vi "Init.vi"(7 "Section Name":refnum<class "Section Name.lvclass">, 8 "Error In":errorcluster, 9 "Values":refnum<class "Value.lvclass">[](array[class]), 10 "Keys":refnum<class "Key Name.lvclass">[](array[class]), 11 "reference in":refnum<class "Dummy Entry.lvclass">) -> (0 "Error Out":errorcluster, 3 "reference out":refnum<class "Dummy Entry.lvclass">)   [LabVIEW 2024, in "Electronic Datasheet.lvlib" / "Dummy Entry.lvclass"]
uses:
  Dummy Entry.lvclass
  Dummy Entry.lvclass/Dummy Entry.ctl
  Object Type/Object Type Base.lvclass
  OD Entry/OD Entry.lvclass
  D:/git/EDS-File-Viewer/Core/OD Entry/OD Entry.lvclass
  D:/git/EDS-File-Viewer/Core/Dummy Entry/Dummy Entry.lvclass
  Section Name/Section Name.lvclass
  Value/Value.lvclass
  Keyname/Key Name.lvclass
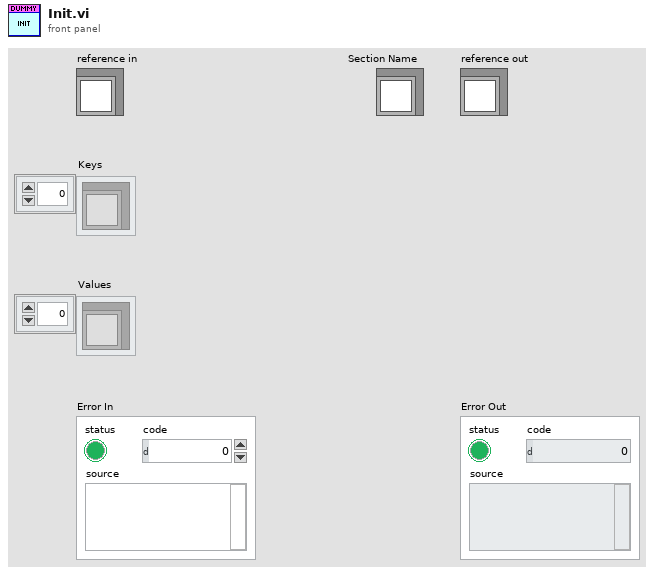
[diagram p1: front panel]
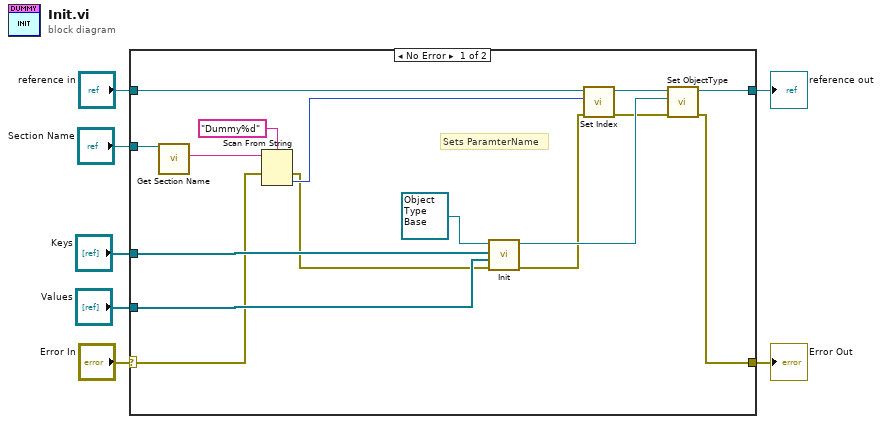
[diagram p0: block diagram]
diagram:
  n1 = case shown="No Error" "Error In" {
    selector: "Error In" -> [w9 w25]
    tunnel: [w18 w25] -> w6
    tunnel: [w20 w24] -> w4
    tunnel: "reference in" -> [w17 w24]
    tunnel: "Keys" -> [w23 _]
    tunnel: "Values" -> [w22 _]
    tunnel: "Section Name" -> [w13 _]
    frame No Error {
      # "Sets ParamterName"
      n2 = call "Get Section Name.vi"("Section Name in"=w13) -> ("Section Name"=w12:string)  [unwired: 9 in, 1 out]
      n3 = Scan From String(format string="Dummy%d", input string=w12, error in=w9) -> (error out=w8:errorcluster, output 1=w10:u16)  [unwired: 2 in, 2 out]
      n4 = call-dynamic "Init.vi"("error in"=w8, "Values"=w22, "Keys"=w23, "Object Type in"=refnum<class "Object Type Base.lvclass"> refnum ("Electronic Datasheet.lvlib:Object Type Base.lvclass")) -> ("error out"=w15:errorcluster, "Object Type out"=w19:refnum<class "Object Type Base.lvclass">)  [unwired: 6 in]
      n5 = call "Set Index.vi"("Error In"=w15, "Index"=w10, "reference in"=w17) -> ("Error Out"=w14:errorcluster, "reference out"=w16:refnum<class "Dummy Entry.lvclass">)  [unwired: 7 in]
      n6 = call "Set ObjectType.vi"("Error In"=w14, "ObjectType"=w19, "reference in"=w16) -> ("Error Out"=w18:errorcluster, "reference out"=w20:refnum<class "Dummy Entry.lvclass">)  [unwired: 7 in]
    }
    frame Error {
    }
  }
  "Error Out" <- w6
  "reference out" <- w4
